vi "Convert TimeString To TimeStamp(HH_MM_SS).vi"() -> ()   [LabVIEW 2015]
uses:
  <vilib>/Utility/miscctls.llb/LVDateTimeRec.ctl
panel:
  out "time stamp":timestamp
  in  "时间字符串（H:MM）":string
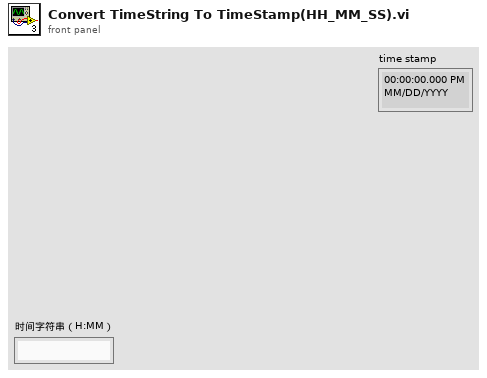
[diagram p1: front panel]
types:
  T1 = typedef "LVDateTimeRec.ctl" = cluster{"fractional second":dbl, "second":i32, "minute":i32, "hour":i32, "day of month":i32, "month":i32, "year":i32, "day of week":i32, "day of year":i32, "DST":i32}
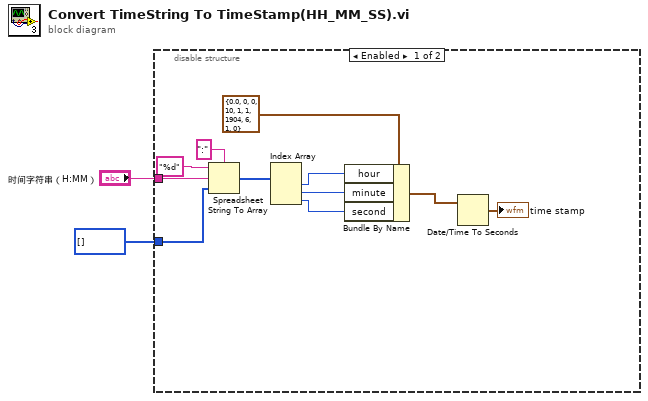
[diagram p0: block diagram]
diagram:
  n1 = disable-structure shown="Enabled" {
    disable-tunnel: "时间字符串（H:MM）" -> [w9 _]
    disable-tunnel: i32[] [] -> [w10 _]
    frame Enabled {
      n2 = Spreadsheet String To Array(delimiter (Tab)=":", format string="%d", spreadsheet string=w9, array type (2D Dbl)=w10) -> (array=w6:i32[])
      n3 = Index Array(array=w6) -> (element #1=w5:i32, element #2=w4:i32, element #3=w3:i32)  [unwired: 3 in]
      n4 = Bundle By Name(cluster=T1 {"fractional second"=0.0, "second"=0, "minute"=0, "hour"=10, "day of month"=1, "month"=1, "year"=1904, "day of week"=6, "day of year"=1, "DST"=0} ("date time rec"), "hour"=w5, "minute"=w4, "second"=w3) -> (w13:T1)
      n5 = Date/Time To Seconds(2:w13) -> (0:→"time stamp":timestamp)  [unwired: 1 in]
    }
    frame Disabled {
    }
  }
